vi "BK Precision 9132B Output DC Volts.vi"() -> ()   [LabVIEW 2017]
doc: "This example shows how to configure the instrument's output voltage level and over voltage protection. The actual voltage level and actual current level are returned."
uses:
  <instrlib>/BK Precision 913XX/BK Precision 913XX.lvlib
panel:
  in  "Voltage Limit (6.000 V)":dbl=36.0 min=0.0 max=66.0 step=0.001 format="%.3g"
  in  "Enable OVP (T: Enable)":bool=TRUE
  in  "Channel (3:3)":u16(ring)=1 items=["1"=1, "2"=2, "3"=3]
  in  "Current Limit (0.0 A)":dbl min=0.0 max=25.0 step=1.0 format="%.3f"
  in  "Stop Output 3":bool
  out "Actual Current Level (A)":dbl format="%.4g"
  out "Actual Power Level (W)":dbl format="%.4g"
  out "Actual Voltage Level (V)":dbl format="%.4g"
  in  "Voltage Level (0.0 V)":dbl format="%.3g"
  in  "VISA resource name":refnum<visa-resource-name>
  in  "Voltage Limit (36.000 V)":dbl=36.0 min=0.0 max=66.0 step=0.001 format="%.3g"
  in  "Enable OVP (T: Enable)":bool=TRUE
  in  "Channel (2:2)":u16(ring)=1 items=["1"=1, "2"=2, "3"=3]
  in  "Current Limit (0.0 A)":dbl min=0.0 max=25.0 step=1.0 format="%.3f"
  in  "Stop Output 2":bool
  out "Actual Current Level (A)":dbl format="%.4g"
  out "Actual Power Level (W)":dbl format="%.4g"
  out "Actual Voltage Level (V)":dbl format="%.4g"
  in  "Voltage Level (0.0 V)":dbl format="%.3g"
  in  "VISA resource name":refnum<visa-resource-name>
  out "Actual Power Level (W)":dbl format="%.4g"
  out "Actual Voltage Level (V)":dbl format="%.4g"
  out "Actual Current Level (A)":dbl format="%.4g"
  in  "Voltage Limit (36.000 V)":dbl=36.0 min=0.0 max=66.0 step=0.001 format="%.3g"
  in  "Enable OVP (T: Enable)":bool=TRUE
  in  "Channel (1:1)":u16(ring)=1 items=["1"=1, "2"=2, "3"=3]
  in  "Current Limit (0.0 A)":dbl min=0.0 max=25.0 step=1.0 format="%.3f"
  in  "Voltage Level (0.0 V)":dbl format="%.3g"
  in  "Stop Output":bool
  in  "VISA resource name":refnum<visa-resource-name>
  # "C H A N N E L  0 1"
  # "V"
  # "Over Voltage Protection"
  # "V"
  # "C H A N N E L  0 2"
  # "Over Voltage Protection"
  # "C H A N N E L  0 3"
  # "Over Voltage Protection"
  # "(c) 2015 B&K Precision Corporation.  ALL RIGHTS RESERVED."
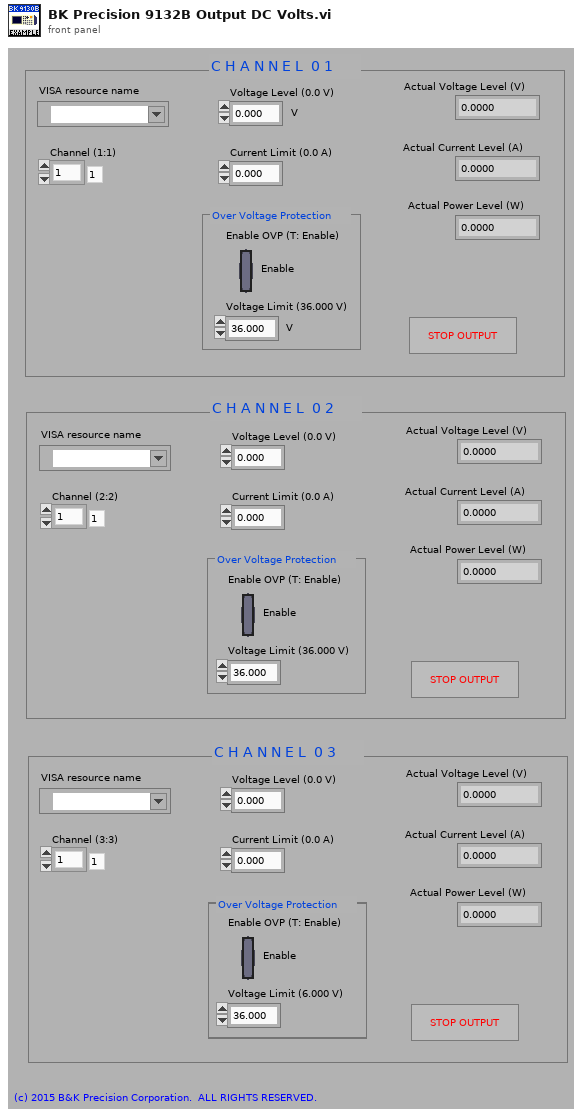
[diagram p1: front panel]
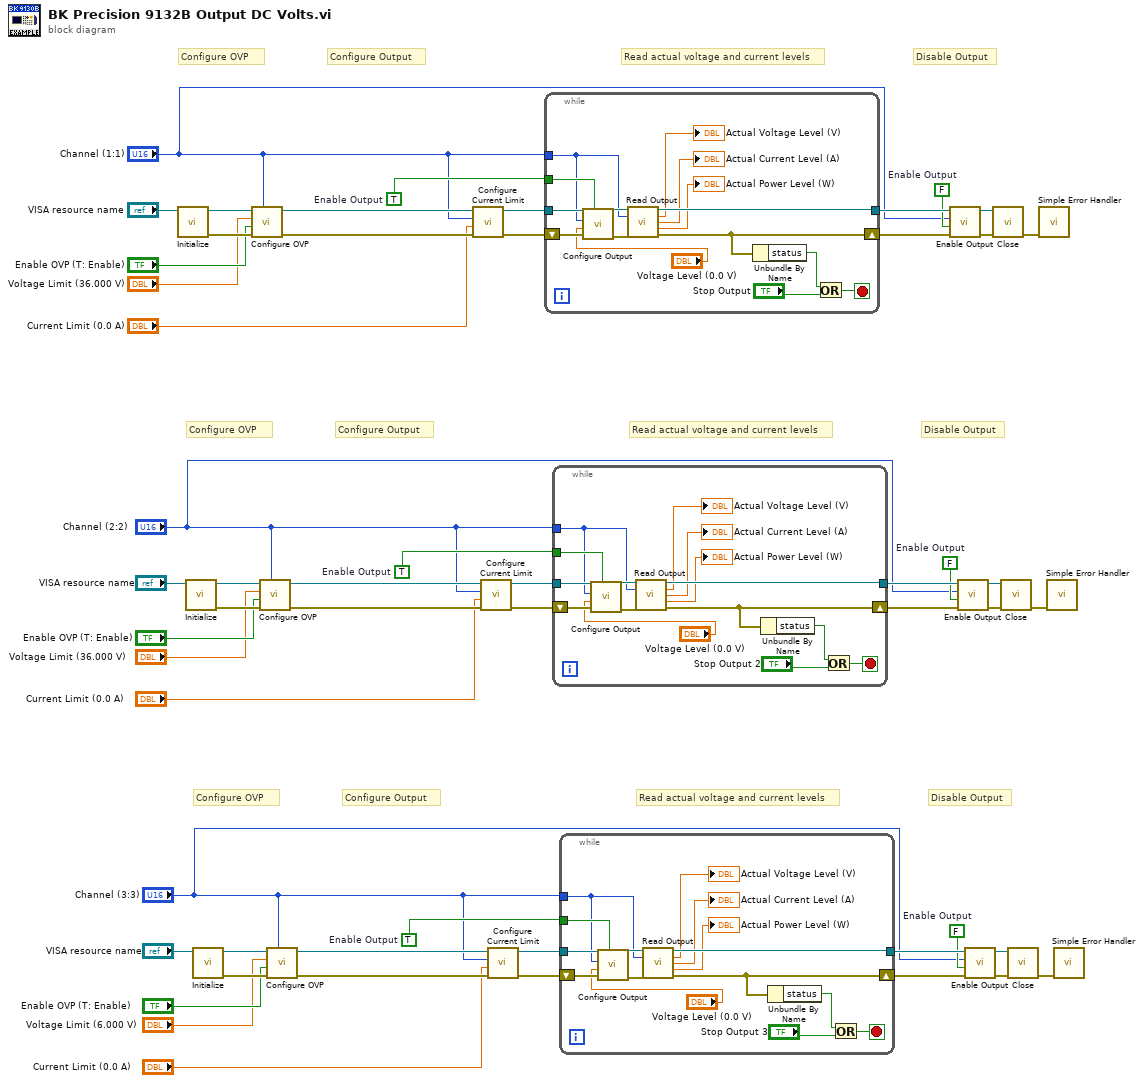
[diagram p0: block diagram]
diagram:
  w2 = TRUE  # Enable Output
  w3 = FALSE  # Enable Output
  w20 = TRUE  # Enable Output
  w21 = FALSE  # Enable Output
  w38 = TRUE  # Enable Output
  w39 = FALSE  # Enable Output
  # "Disable Output"
  # "Read actual voltage and current levels"
  # "Configure Output"
  # "Configure OVP"
  # "Disable Output"
  # "Read actual voltage and current levels"
  # "Configure Output"
  # "Configure OVP"
  # "Disable Output"
  # "Read actual voltage and current levels"
  # "Configure Output"
  # "Configure OVP"
  n1 = call <instrlib>:"Initialize.vi"("VISA resource name"="VISA resource name") -> ("error out"=w52:errorcluster, "VISA resource name out"=w51:refnum<visa-resource-name>)  [unwired: 9 in]
  n2 = call <instrlib>:"Initialize.vi"("VISA resource name"="VISA resource name") -> ("error out"=w34:errorcluster, "VISA resource name out"=w33:refnum<visa-resource-name>)  [unwired: 9 in]
  n3 = call <instrlib>:"Initialize.vi"("VISA resource name"="VISA resource name") -> ("error out"=w16:errorcluster, "VISA resource name out"=w15:refnum<visa-resource-name>)  [unwired: 9 in]
  n4 = call <instrlib>:"Configure OVP.vi"("Channel (1:1)"="Channel (1:1)", "error in (no error)"=w52, "Enable OVP (T: Enable)"="Enable OVP (T: Enable)", "Voltage Limit (36.000 V)"="Voltage Limit (36.000 V)", "VISA resource name"=w51) -> ("error out"=w49:errorcluster, "VISA resource name out"=w50:refnum<visa-resource-name>)  [unwired: 5 in]
  n5 = call <instrlib>:"Configure OVP.vi"("Channel (1:1)"="Channel (2:2)", "error in (no error)"=w34, "Enable OVP (T: Enable)"="Enable OVP (T: Enable)", "Voltage Limit (36.000 V)"="Voltage Limit (36.000 V)", "VISA resource name"=w33) -> ("error out"=w31:errorcluster, "VISA resource name out"=w32:refnum<visa-resource-name>)  [unwired: 5 in]
  n6 = call <instrlib>:"Configure OVP.vi"("Channel (1:1)"="Channel (3:3)", "error in (no error)"=w16, "Enable OVP (T: Enable)"="Enable OVP (T: Enable)", "Voltage Limit (36.000 V)"="Voltage Limit (6.000 V)", "VISA resource name"=w15) -> ("error out"=w13:errorcluster, "VISA resource name out"=w14:refnum<visa-resource-name>)  [unwired: 5 in]
  n7 = call <instrlib>:"Configure Current Limit.vi"("error in (no error)"=w49, "Current Limit (0.0 A)"="Current Limit (0.0 A)", "Channel (1:1)"="Channel (1:1)", "VISA resource name"=w50) -> ("error out"=w45:errorcluster, "VISA resource name out"=w44:refnum<visa-resource-name>)  [unwired: 6 in]
  n8 = call <instrlib>:"Configure Current Limit.vi"("error in (no error)"=w31, "Current Limit (0.0 A)"="Current Limit (0.0 A)", "Channel (1:1)"="Channel (2:2)", "VISA resource name"=w32) -> ("error out"=w27:errorcluster, "VISA resource name out"=w26:refnum<visa-resource-name>)  [unwired: 6 in]
  n9 = call <instrlib>:"Configure Current Limit.vi"("error in (no error)"=w13, "Current Limit (0.0 A)"="Current Limit (0.0 A)", "Channel (1:1)"="Channel (3:3)", "VISA resource name"=w14) -> ("error out"=w9:errorcluster, "VISA resource name out"=w8:refnum<visa-resource-name>)  [unwired: 6 in]
  n10 = while {
    tunnel: w44 -> [w59]
    tunnel: [w65] -> w48
    shift-right: [w66] -> w43
    shift-left: w45 -> [w61]
    tunnel: "Channel (1:1)" -> [w55]
    tunnel: w38 -> [w57]
    stop <- w69 stop-if-true
    n11 = call <instrlib>:"Configure Output.vi"("Enable Channel Output (F: False)"=w57, "error in (no error)"=w61, "Voltage Level (0.0 V)"="Voltage Level (0.0 V)", "Channel (1:1)"=w55, "VISA resource name"=w59) -> ("error out"=w60:errorcluster, "VISA resource name out"=w58:refnum<visa-resource-name>)  [unwired: 5 in]
    n12 = call <instrlib>:"Read Output.vi"("VISA resource name"=w58, "Channel (1:Channel 1)"=w55, "error in (no error)"=w60) -> ("VISA resource name out"=w65:refnum<visa-resource-name>, "Actual Voltage Level (V)"=→"Actual Voltage Level (V)":dbl, "Actual Current Level (A)"=→"Actual Current Level (A)":dbl, "Actual Power Level (W)"=→"Actual Power Level (W)":dbl, "error out"=w66:errorcluster)  [unwired: 8 in]
    n13 = Unbundle By Name(w66) -> ("status"=w67:bool)
    n14 = Or(x=w67, y="Stop Output") -> (x .or. y?=w69:bool)
  }
  n15 = while {
    tunnel: w26 -> [w74]
    tunnel: [w80] -> w30
    shift-right: [w81] -> w25
    shift-left: w27 -> [w76]
    tunnel: "Channel (2:2)" -> [w70]
    tunnel: w20 -> [w72]
    stop <- w84 stop-if-true
    n16 = call <instrlib>:"Configure Output.vi"("Enable Channel Output (F: False)"=w72, "error in (no error)"=w76, "Voltage Level (0.0 V)"="Voltage Level (0.0 V)", "Channel (1:1)"=w70, "VISA resource name"=w74) -> ("error out"=w75:errorcluster, "VISA resource name out"=w73:refnum<visa-resource-name>)  [unwired: 5 in]
    n17 = call <instrlib>:"Read Output.vi"("VISA resource name"=w73, "Channel (1:Channel 1)"=w70, "error in (no error)"=w75) -> ("VISA resource name out"=w80:refnum<visa-resource-name>, "Actual Voltage Level (V)"=→"Actual Voltage Level (V)":dbl, "Actual Current Level (A)"=→"Actual Current Level (A)":dbl, "Actual Power Level (W)"=→"Actual Power Level (W)":dbl, "error out"=w81:errorcluster)  [unwired: 8 in]
    n18 = Unbundle By Name(w81) -> ("status"=w82:bool)
    n19 = Or(x=w82, y="Stop Output 2") -> (x .or. y?=w84:bool)
  }
  n20 = while {
    tunnel: w8 -> [w89]
    tunnel: [w95] -> w12
    shift-right: [w96] -> w7
    shift-left: w9 -> [w91]
    tunnel: "Channel (3:3)" -> [w85]
    tunnel: w2 -> [w87]
    stop <- w99 stop-if-true
    n21 = call <instrlib>:"Configure Output.vi"("Enable Channel Output (F: False)"=w87, "error in (no error)"=w91, "Voltage Level (0.0 V)"="Voltage Level (0.0 V)", "Channel (1:1)"=w85, "VISA resource name"=w89) -> ("error out"=w90:errorcluster, "VISA resource name out"=w88:refnum<visa-resource-name>)  [unwired: 5 in]
    n22 = call <instrlib>:"Read Output.vi"("VISA resource name"=w88, "Channel (1:Channel 1)"=w85, "error in (no error)"=w90) -> ("VISA resource name out"=w95:refnum<visa-resource-name>, "Actual Voltage Level (V)"=→"Actual Voltage Level (V)":dbl, "Actual Current Level (A)"=→"Actual Current Level (A)":dbl, "Actual Power Level (W)"=→"Actual Power Level (W)":dbl, "error out"=w96:errorcluster)  [unwired: 8 in]
    n23 = Unbundle By Name(w96) -> ("status"=w97:bool)
    n24 = Or(x=w97, y="Stop Output 3") -> (x .or. y?=w99:bool)
  }
  n25 = call <instrlib>:"Enable Output.vi"("error in (no error)"=w43, "Enable Output (F: False)"=w39, "Channel (1:1)"="Channel (1:1)", "VISA resource name"=w48) -> ("error out"=w46:errorcluster, "VISA resource name out"=w47:refnum<visa-resource-name>)  [unwired: 6 in]
  n26 = call <instrlib>:"Enable Output.vi"("error in (no error)"=w25, "Enable Output (F: False)"=w21, "Channel (1:1)"="Channel (2:2)", "VISA resource name"=w30) -> ("error out"=w28:errorcluster, "VISA resource name out"=w29:refnum<visa-resource-name>)  [unwired: 6 in]
  n27 = call <instrlib>:"Enable Output.vi"("error in (no error)"=w7, "Enable Output (F: False)"=w3, "Channel (1:1)"="Channel (3:3)", "VISA resource name"=w12) -> ("error out"=w10:errorcluster, "VISA resource name out"=w11:refnum<visa-resource-name>)  [unwired: 6 in]
  n28 = call <instrlib>:"Close.vi"("error in (no error)"=w46, "VISA resource name"=w47) -> ("error out"=w53:errorcluster)  [unwired: 9 in]
  n29 = call <instrlib>:"Close.vi"("error in (no error)"=w28, "VISA resource name"=w29) -> ("error out"=w35:errorcluster)  [unwired: 9 in]
  n30 = call <instrlib>:"Close.vi"("error in (no error)"=w10, "VISA resource name"=w11) -> ("error out"=w17:errorcluster)  [unwired: 9 in]
  n31 = call <vilib>:"Simple Error Handler.vi"("error in (no error)"=w53) -> ()  [unwired: 4 in, 5 out]
  n32 = call <vilib>:"Simple Error Handler.vi"("error in (no error)"=w35) -> ()  [unwired: 4 in, 5 out]
  n33 = call <vilib>:"Simple Error Handler.vi"("error in (no error)"=w17) -> ()  [unwired: 4 in, 5 out]
